vi "AR Model Estimation.vi"() -> ()   [LabVIEW 2023]
doc: "This example shows how to obtain AR model parameters of a univariate time series using the TSA AR Modeling VI.\n\n<b>Instructions:</b>\n1) Run this VI.\n2) Set the coefficients for the IIR filter.\n3) Observe the detected coefficients from AR modeling."
uses:
  <vilib>/Analysis/3filter.llb/IIR Filter (DBL).vi
  <vilib>/addons/Time Series Analysis/Modeling and Prediction.llb/TSA AR Modeling (Array).vi
  <vilib>/addons/_Advanced Signal Processing/NI_AdvSigProcTSA.lvlib
  <vilib>/Analysis/NI_AALBase.lvlib
panel:
  out "Time Series from the Simulated System":dbl[](graph)
  in  "stop":bool
  out "Estimated AR coefficients":dbl[](array[numeric])
  in  "Reverse coefficients":dbl[](array[numeric])=[1.0, 1.5, 0.7, 0.1]
  out "AR Coefficients":dbl[][](graph)
  in  "Method":u16(ring) items=["Forward-Backward", "Least-Squares", "Yule-Walker", "Burg-Lattice", "Geometric-Lattice"]
  # "Overview: Shows how to obtain AR model parameters of a univariate time series using the TSA AR Modeling VI.\nRequirements: LabVIEW Full Development System, Advanced Signal Processing Toolkit\nInstructions: \n1. Run this VI.\n2. Set the coefficients for the IIR filter.\n3. Observe the detected coefficients from AR modeling.\n4. Click Stop to stop the VI."
  # "Simulated System (IIR Filter)"
  # "The first element of the Reverse coefficients must be 1."
  # "Forward coefficients = [1]"
  # "AR Modeling Settings"
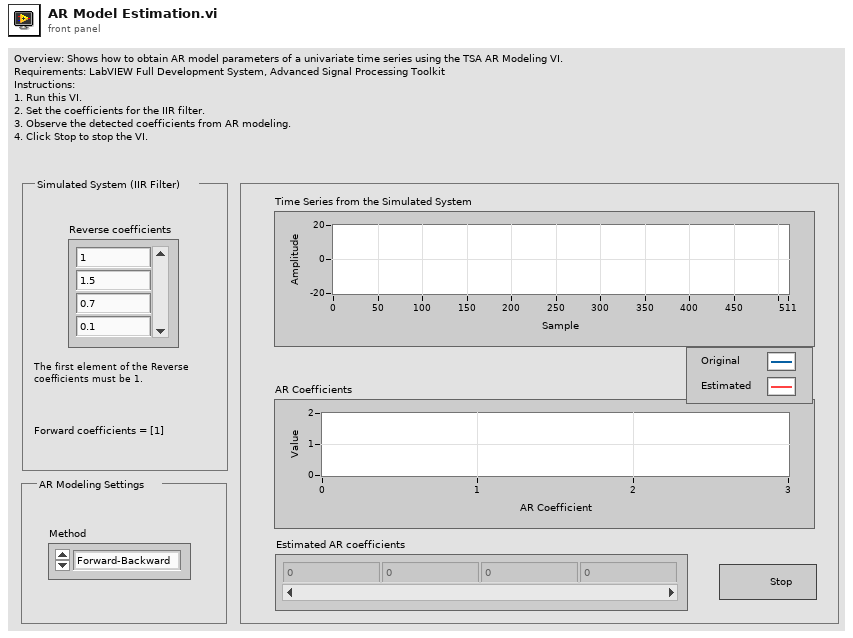
[diagram p1: front panel]
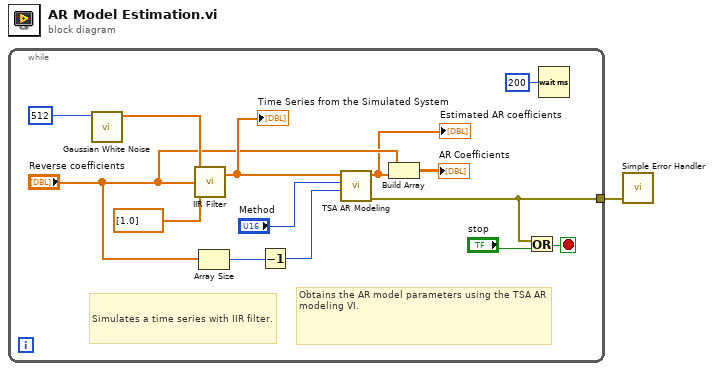
[diagram p0: block diagram]
diagram:
  n1 = while {
    tunnel: [w2] -> w1
    stop <- w5 stop-if-true
    # "Obtains the AR model parameters using the TSA AR modeling VI."
    # "Simulates a time series with IIR filter."
    n2 = call <vilib>:"Gaussian White Noise.vi"("samples"=512) -> ("Gaussian noise pattern"=w15:dbl[])  [unwired: 9 in, 1 out]
    n3 = call-poly <vilib>:"IIR Filter.vi"("Forward Coefficients"=dbl[] [1.0], "Reverse Coefficients"="Reverse coefficients", "X"=w15) -> ("Filtered X"=w13:dbl[])  [unwired: 1 in, 1 out]
    "Time Series from the Simulated System" <- w13
    n4 = Array Size(array="Reverse coefficients") -> (size(s)=w8:i32)
    n5 = Decrement(x=w8) -> (x-1=w7:i32)
    n6 = call-poly <vilib>:"TSA AR Modeling.vi"("AR order"=w7, "AR method"="Method", "Xt"=w13) -> ("error out"=w2:errorcluster, "AR coefficients"=w3:dbl[])  [unwired: 1 in, 6 out]
    "Estimated AR coefficients" <- w3
    n7 = Build Array("Reverse coefficients", w3) -> (→"AR Coefficients":dbl[][])
    n8 = Or(x=w2, y="stop") -> (x .or. y?=w5:bool)
    n9 = Wait (ms)(milliseconds to wait=u32 200 ("millisecond multiple")) -> ()  [unwired: 1 out]
  }
  n10 = call <vilib>:"Simple Error Handler.vi"("error in (no error)"=w1) -> ()  [unwired: 1 in, 8 out]
